vi "Method.vi"(4 "Value B":refnum<class "Abs_Numeric.lvclass">, 5 "Value A":refnum<class "Abs_Double Float.lvclass">) -> (1 "Result":refnum<class "Abs_Boolean.lvclass">)   [LabVIEW 2021, in "Less_DBL.lvclass"]
uses:
  Less_DBL.lvclass
  Abs_Types/Double Float/Abs_Double Float.lvclass
  Abs_Types/Boolean/Abs_Boolean.lvclass
  Abs_Types/Numeric/Abs_Numeric.lvclass
  C:/Users/Tim/Documents/GitHub/LV_Abstract/Source/Functions/Support/Compare/Two Term/DBL/AbsComp_Two Term_DBL.lvclass
  C:/Users/Tim/Documents/GitHub/LV_Abstract/Source/Abs_Types/Boolean/Abs_Boolean.lvclass
  Support/Compare/Two Term/DBL/AbsComp_Two Term_DBL.lvclass/AbsComp_Two Term_DBL.ctl
  Support/Compare/Two Term/DBL/Properties/Write Numeric A.vi
  Support/Compare/Two Term/DBL/Properties/Write Numeric B.vi
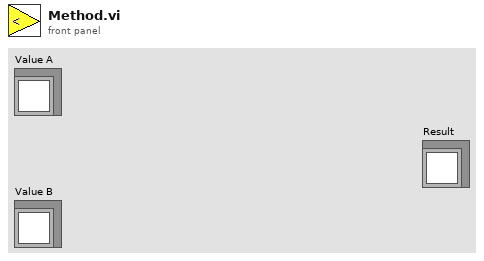
[diagram p1: front panel]
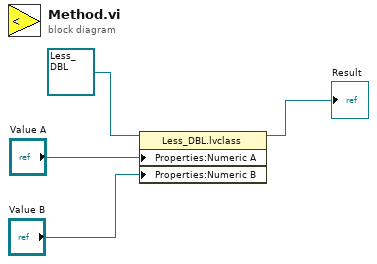
[diagram p0: block diagram]
diagram:
  n1 = property class="Less_DBL.lvclass"(reference=refnum<class "Less_DBL.lvclass"> refnum ("Greater 0_U64.lvclass"), "Properties:Numeric A"="Value A", "Properties:Numeric B"="Value B") -> (reference out=→"Result":refnum<class "Less_DBL.lvclass">)  [unwired: 1 in, 1 out]
